vi "Test Clahe Mono Array.vi"(8 "error in (no error)":errorcluster, 11 "Test Case In":refnum<class "01_Image.lvclass">) -> (0 "error out":errorcluster, 3 "Test Case Out":refnum<class "01_Image.lvclass">)   [LabVIEW 2020, in "test.lvlib" / "01_Image.lvclass"]
uses:
  01_Image.lvclass
  4993e8ee-a06a-463a-9684-69129f64d5ce.vi
  image/CLAHE/CLAHE.lvclass
  image/image.lvlib
  image/New Image (Greyscale Preallocated).vi
panel:
  out "data value":u8[][](array[numeric])
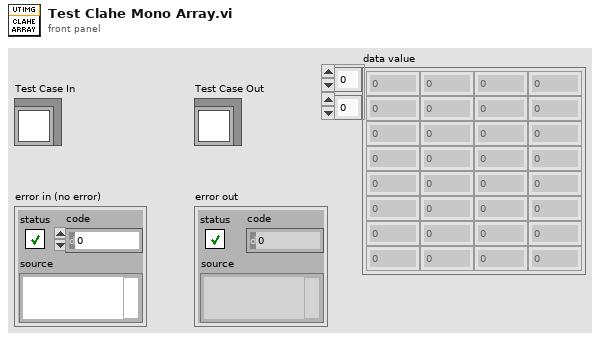
[diagram p1: front panel]
types:
  T1 = typedef "image.lvlib/Greyscale Image.ctl" = refnum<data-value>
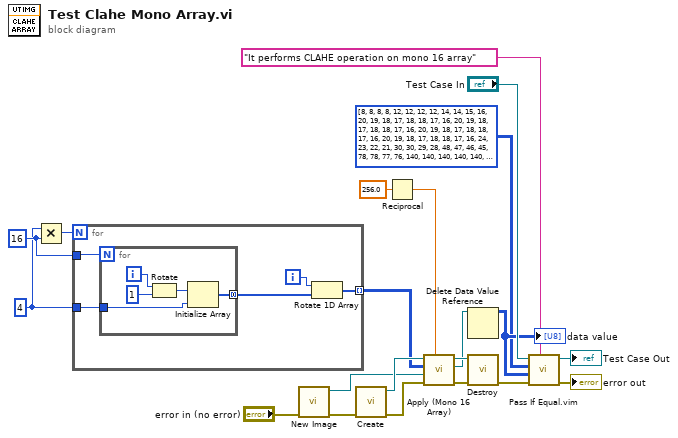
[diagram p0: block diagram]
diagram:
  w8 = 4 ("dimension size")
  w10 = 16
  n1 = Multiply(x=w8, y=w10) -> (x*y=w9:i32)
  n2 = for {
    N: w9 -> [_]
    tunnel: [w24] -> w7 mode=indexing
    tunnel: w10 -> [w23]
    tunnel: w8 -> [w22]
    i -> [w25]
    n3 = for {
      N: w23 -> [_]
      tunnel: [w28] -> w26 mode=concatenating
      tunnel: w22 -> [w27]
      i -> [w31]
      n4 = Rotate(1:u16 1 ("x"), 2:w31) -> (0:w29:u16)
      n5 = Initialize Array(w29, w27) -> (w28:u16[])
    }
    n6 = Rotate 1D Array(1:w26, 2:w25) -> (0:w24:u16[])
  }
  n7 = call-poly "New Image.vi"("error in (no error)"="error in (no error)") -> ("error out"=w15:errorcluster, "Greyscale Image"=w16:T1)  [unwired: 9 in]
  n8 = call "Create.vi"("error in (no error)"=w15) -> ("error out"=w14:errorcluster, "CLAHE"=w18:refnum<class "CLAHE.lvclass">)  [unwired: 9 in]
  n9 = Reciprocal(x=256.0 ("Scaling Factor (Default 1/256)")) -> (1/x=w1:dbl)
  n10 = call "Apply (Mono 16 Array).vi"("Scaling Factor (Default 1/256)"=w1, "error in (no error)"=w14, "Destination Image in"=w16, "Mono 16 Image Data"=w7, "CLAHE in"=w18) -> ("error out"=w13:errorcluster, "Destination Image"=w4:T1, "CLAHE"=w17:refnum<class "CLAHE.lvclass">)  [unwired: 4 in]
  n11 = Delete Data Value Reference(data value reference=w4) -> (data value=w3:u8[][])  [unwired: 1 in, 1 out]
  "data value" <- w3
  n12 = call "Destroy.vi"("error in (no error)"=w13, "CLAHE"=w17) -> ("error out"=w12:errorcluster)  [unwired: 9 in]
  n13 = call "Pass If Equal.vim"("Description"="It performs CLAHE operation on mono 16 array", "error in (no error)"=w12, "Actual"=w3, "Expected"=u8[][] [[8, 8, 8, 8, 12, 12, 12, 12, 14, 14, 15, 16, 20, 19, 18, 17, 18, 18, 17, 16, 20, 19, 18, 17, 18, 18, 17, 16, 20, 19, 18, 17, 18, 18, 17, 16, 20, 19, 18, 17, 18, 18, 17, 16, 24, 23, 22, 21, 30, 30, 29, 28, 48, 47, 46, 45, 78, 78, 77, 76, 140, 140, 140, 140], [140, 8, 8, 8, 8, 12, 12, 12, 12, 14, 15, 16, 16, 19, 18, 17, 16, 18, 17, 16, 16, 19, 18, 17, 16, 18, 17, 16, 16, 19, 18, 17, 16, 18, 17, 16, 16, 19, 18, 17, 16, 18, 17, 16, 16, 23, 22, 21, 20, 30, 29, 28, 28, 47, 46, 45, 44, 78, 77, 76, 76, 140, 140, 140], [140, 140, 8, 8, 8, 8, 12, 12, 12, 12, 15, 16, 16, 15, 18, 17, 16, 15, 17, 16, 16, 15, 18, 17, 16, 15, 17, 16, 16, 15, 18, 17, 16, 15, 17, 16, 16, 15, 18, 17, 16, 15, 17, 16, 16, 15, 22, 21, 20, 19, 29, 28, 28, 27, 46, 45, 44, 43, 77, 76, 76, 76, 140, 140], [140, 140, 140, 8, 8, 8, 8, 12, 12, 12, 12, 16, 16, 15, 14, 17, 16, 15, 14, 16, 16, 15, 14, 17, 16, 15, 14, 16, 16, 15, 14, 17, 16, 15, 14, 16, 16, 15, 14, 17, 16, 15, 14, 16, 16, 15, 14, 21, 20, 19, 18, 28, 28, 27, 26, 45, 44, 43, 42, 76, 76, 76, 76, 140], [140, 140, 140, 140, 8, 8, 8, 8, 12, 12, 12, 12, 16, 15, 14, 13, 16, 15, 14, 13, 16, 15, 14, 13, 16, 15, 14, 13, 16, 15, 14, 13, 16, 15, 14, 13, 16, 15, 14, 13, 16, 15, 14, 13, 16, 15, 14, 13, 20, 19, 18, 17, 28, 27, 26, 25, 44, 43, 42, 41, 76, 76, 76, 76], [76, 140, 140, 140, 140, 8, 8, 8, 8, 12, 12, 12, 12, 15, 14, 13, 12, 15, 14, 14, 13, 16, 15, 14, 13, 16, 15, 14, 13, 16, 15, 14, 13, 16, 15, 14, 13, 16, 15, 14, 13, 16, 15, 14, 13, 16, 15, 14, 13, 20, 19, 18, 17, 28, 27, 26, 25, 44, 43, 42, 41, 76, 76, 76], [76, 76, 140, 140, 140, 140, 7, 7, 8, 8, 12, 12, 12, 11, 14, 13, 12, 12, 15, 14, 14, 13, 15, 14, 14, 13, 16, 15, 14, 13, 15, 14, 14, 13, 16, 15, 14, 13, 15, 14, 14, 13, 16, 15, 14, 13, 15, 14, 14, 13, 20, 19, 18, 17, 27, 26, 26, 25, 44, 43, 42, 42, 77, 77], [76, 76, 76, 140, 140, 140, 140, 7, 7, 7, 8, 12, 12, 11, 11, 13, 13, 12, 12, 15, 15, 14, 13, 15, 14, 13, 13, 16, 15, 14, 13, 15, 14, 13, 13, 16, 15, 14, 13, 15, 14, 13, 13, 16, 15, 14, 13, 15, 14, 13, 13, 20, 19, 18, 17, 27, 26, 25, 25, 44, 43, 43, 43, 78], [76, 76, 76, 76, 140, 140, 140, 140, 7, 7, 8, 8, 12, 12, 11, 10, 13, 13, 12, 12, 16, 15, 14, 13, 15, 14, 14, 13, 16, 15, 14, 13, 15, 14, 14, 13, 16, 15, 14, 13, 15, 14, 14, 13, 16, 15, 14, 13, 15, 14, 14, 13, 20, 19, 18, 17, 27, 26, 26, 25, 44, 44, 44, 44], [40, 76, 76, 76, 76, 140, 140, 140, 140, 7, 7, 8, 8, 12, 11, 11, 10, 13, 13, 13, 13, 16, 15, 14, 13, 15, 14, 14, 13, 16, 15, 14, 13, 15, 14, 14, 13, 16, 15, 14, 13, 15, 14, 14, 13, 16, 15, 14, 13, 15, 14, 14, 13, 20, 19, 18, 17, 27, 26, 26, 25, 45, 45, 45], [40, 40, 76, 76, 76, 76, 140, 140, 140, 140, 7, 8, 8, 8, 12, 11, 11, 11, 14, 14, 14, 13, 16, 15, 14, 13, 15, 15, 14, 13, 16, 15, 14, 13, 15, 15, 14, 13, 16, 15, 14, 13, 15, 15, 14, 13, 16, 15, 14, 13, 15, 15, 14, 13, 20, 19, 18, 17, 27, 27, 26, 26, 46, 46], [40, 40, 40, 76, 76, 76, 76, 140, 140, 140, 140, 8, 8, 8, 8, 12, 12, 11, 11, 15, 15, 14, 13, 16, 15, 14, 13, 16, 15, 14, 13, 16, 15, 14, 13, 16, 15, 14, 13, 16, 15, 14, 13, 16, 15, 14, 13, 16, 15, 14, 13, 16, 15, 14, 13, 20, 19, 18, 17, 28, 27, 27, 27, 47], [40, 40, 40, 40, 76, 76, 76, 76, 140, 140, 140, 140, 8, 8, 8, 8, 12, 12, 12, 12, 16, 15, 14, 13, 16, 15, 14, 13, 16, 15, 14, 13, 16, 15, 14, 13, 16, 15, 14, 13, 16, 15, 14, 13, 16, 15, 14, 13, 16, 15, 14, 13, 16, 15, 14, 13, 20, 19, 18, 17, 28, 28, 28, 28], [21, 41, 41, 41, 41, 76, 76, 76, 76, 140, 140, 140, 140, 8, 8, 8, 8, 12, 12, 12, 12, 15, 14, 13, 12, 15, 14, 14, 13, 16, 15, 14, 13, 16, 15, 14, 13, 16, 15, 14, 13, 16, 15, 14, 13, 16, 15, 14, 13, 16, 15, 14, 13, 16, 15, 14, 13, 20, 19, 18, 17, 28, 28, 28], [22, 22, 42, 42, 42, 42, 77, 77, 76, 76, 140, 140, 140, 140, 7, 7, 8, 8, 12, 12, 12, 11, 14, 13, 12, 12, 15, 14, 14, 13, 15, 14, 14, 13, 16, 15, 14, 13, 15, 14, 14, 13, 16, 15, 14, 13, 15, 14, 14, 13, 16, 15, 14, 13, 15, 14, 14, 13, 20, 19, 18, 18, 29, 29], [23, 23, 23, 43, 43, 43, 42, 77, 77, 77, 76, 140, 140, 140, 140, 7, 7, 7, 8, 12, 12, 11, 11, 13, 13, 12, 12, 15, 15, 14, 13, 15, 14, 13, 13, 16, 15, 14, 13, 15, 14, 13, 13, 16, 15, 14, 13, 15, 14, 13, 13, 16, 15, 14, 13, 15, 14, 13, 13, 20, 19, 19, 19, 30], [24, 24, 24, 24, 44, 44, 43, 42, 77, 77, 76, 76, 140, 140, 140, 140, 7, 7, 8, 8, 12, 12, 11, 10, 13, 13, 12, 12, 16, 15, 14, 13, 15, 14, 14, 13, 16, 15, 14, 13, 15, 14, 14, 13, 16, 15, 14, 13, 15, 14, 14, 13, 16, 15, 14, 13, 15, 14, 14, 13, 20, 20, 20, 20], [13, 25, 25, 25, 25, 44, 44, 43, 42, 77, 77, 76, 76, 140, 140, 140, 140, 7, 7, 8, 8, 12, 11, 11, 10, 13, 13, 13, 13, 16, 15, 14, 13, 15, 14, 14, 13, 16, 15, 14, 13, 15, 14, 14, 13, 16, 15, 14, 13, 15, 14, 14, 13, 16, 15, 14, 13, 15, 14, 14, 13, 21, 21, 21], [14, 14, 26, 26, 26, 25, 44, 44, 43, 42, 77, 76, 76, 76, 140, 140, 140, 140, 7, 8, 8, 8, 12, 11, 11, 11, 14, 14, 14, 13, 16, 15, 14, 13, 15, 15, 14, 13, 16, 15, 14, 13, 15, 15, 14, 13, 16, 15, 14, 13, 15, 15, 14, 13, 16, 15, 14, 13, 15, 15, 14, 14, 22, 22], [15, 15, 15, 27, 27, 26, 25, 44, 44, 43, 42, 76, 76, 76, 76, 140, 140, 140, 140, 8, 8, 8, 8, 12, 12, 11, 11, 15, 15, 14, 13, 16, 15, 14, 13, 16, 15, 14, 13, 16, 15, 14, 13, 16, 15, 14, 13, 16, 15, 14, 13, 16, 15, 14, 13, 16, 15, 14, 13, 16, 15, 15, 15, 23], [16, 16, 16, 16, 28, 27, 26, 25, 44, 43, 42, 41, 76, 76, 76, 76, 140, 140, 140, 140, 8, 8, 8, 8, 12, 12, 12, 12, 16, 15, 14, 13, 16, 15, 14, 13, 16, 15, 14, 13, 16, 15, 14, 13, 16, 15, 14, 13, 16, 15, 14, 13, 16, 15, 14, 13, 16, 15, 14, 13, 16, 16, 16, 16], [9, 17, 17, 17, 17, 28, 27, 26, 25, 44, 43, 42, 41, 76, 76, 76, 76, 140, 140, 140, 140, 8, 8, 8, 8, 12, 12, 12, 12, 15, 14, 13, 12, 15, 14, 14, 13, 16, 15, 14, 13, 16, 15, 14, 13, 16, 15, 14, 13, 16, 15, 14, 13, 16, 15, 14, 13, 16, 15, 14, 13, 16, 16, 16], [10, 10, 18, 18, 18, 17, 27, 26, 26, 25, 44, 43, 42, 42, 77, 77, 76, 76, 140, 140, 140, 140, 7, 7, 8, 8, 12, 12, 12, 11, 14, 13, 12, 12, 15, 14, 14, 13, 15, 14, 14, 13, 16, 15, 14, 13, 15, 14, 14, 13, 16, 15, 14, 13, 15, 14, 14, 13, 16, 15, 14, 14, 17, 17], [11, 11, 11, 19, 19, 18, 17, 27, 26, 25, 25, 44, 43, 43, 42, 77, 77, 77, 76, 140, 140, 140, 140, 7, 7, 7, 8, 12, 12, 11, 11, 13, 13, 12, 12, 15, 15, 14, 13, 15, 14, 13, 13, 16, 15, 14, 13, 15, 14, 13, 13, 16, 15, 14, 13, 15, 14, 13, 13, 16, 15, 15, 15, 18], [12, 12, 12, 12, 20, 19, 18, 17, 27, 26, 26, 25, 44, 44, 43, 42, 77, 77, 76, 76, 140, 140, 140, 140, 7, 7, 8, 8, 12, 12, 11, 10, 13, 13, 12, 12, 16, 15, 14, 13, 15, 14, 14, 13, 16, 15, 14, 13, 15, 14, 14, 13, 16, 15, 14, 13, 15, 14, 14, 13, 16, 16, 16, 16], [9, 13, 13, 13, 13, 20, 19, 18, 17, 27, 26, 26, 25, 44, 44, 43, 42, 77, 77, 76, 76, 140, 140, 140, 140, 7, 7, 8, 8, 12, 11, 11, 10, 13, 13, 13, 13, 16, 15, 14, 13, 15, 14, 14, 13, 16, 15, 14, 13, 15, 14, 14, 13, 16, 15, 14, 13, 15, 14, 14, 13, 17, 17, 17], [10, 10, 14, 14, 14, 13, 20, 19, 18, 17, 27, 27, 26, 25, 44, 44, 43, 42, 77, 76, 76, 76, 140, 140, 140, 140, 7, 8, 8, 8, 12, 11, 11, 11, 14, 14, 14, 13, 16, 15, 14, 13, 15, 15, 14, 13, 16, 15, 14, 13, 15, 15, 14, 13, 16, 15, 14, 13, 15, 15, 14, 14, 18, 18], [11, 11, 11, 15, 15, 14, 13, 20, 19, 18, 17, 28, 27, 26, 25, 44, 44, 43, 42, 76, 76, 76, 76, 140, 140, 140, 140, 8, 8, 8, 8, 12, 12, 11, 11, 15, 15, 14, 13, 16, 15, 14, 13, 16, 15, 14, 13, 16, 15, 14, 13, 16, 15, 14, 13, 16, 15, 14, 13, 16, 15, 15, 15, 19], [12, 12, 12, 12, 16, 15, 14, 13, 20, 19, 18, 17, 28, 27, 26, 25, 44, 43, 42, 41, 76, 76, 76, 76, 140, 140, 140, 140, 8, 8, 8, 8, 12, 12, 12, 12, 16, 15, 14, 13, 16, 15, 14, 13, 16, 15, 14, 13, 16, 15, 14, 13, 16, 15, 14, 13, 16, 15, 14, 13, 16, 16, 16, 16], [9, 13, 13, 13, 13, 16, 15, 14, 13, 20, 19, 18, 17, 28, 27, 26, 25, 44, 43, 42, 41, 76, 76, 76, 76, 140, 140, 140, 140, 8, 8, 8, 8, 12, 12, 12, 12, 15, 14, 13, 12, 15, 14, 14, 13, 16, 15, 14, 13, 16, 15, 14, 13, 16, 15, 14, 13, 16, 15, 14, 13, 16, 16, 16], [10, 10, 14, 14, 14, 13, 15, 14, 14, 13, 20, 19, 18, 17, 27, 26, 26, 25, 44, 43, 42, 42, 77, 77, 76, 76, 140, 140, 140, 140, 7, 7, 8, 8, 12, 12, 12, 11, 14, 13, 12, 12, 15, 14, 14, 13, 15, 14, 14, 13, 16, 15, 14, 13, 15, 14, 14, 13, 16, 15, 14, 14, 17, 17], [11, 11, 11, 15, 15, 14, 13, 15, 14, 13, 13, 20, 19, 18, 17, 27, 26, 25, 25, 44, 43, 43, 42, 77, 77, 77, 76, 140, 140, 140, 140, 7, 7, 7, 8, 12, 12, 11, 11, 13, 13, 12, 12, 15, 15, 14, 13, 15, 14, 13, 13, 16, 15, 14, 13, 15, 14, 13, 13, 16, 15, 15, 15, 18], [12, 12, 12, 12, 16, 15, 14, 13, 15, 14, 14, 13, 20, 19, 18, 17, 27, 26, 26, 25, 44, 44, 43, 42, 77, 77, 76, 76, 140, 140, 140, 140, 7, 7, 8, 8, 12, 12, 11, 10, 13, 13, 12, 12, 16, 15, 14, 13, 15, 14, 14, 13, 16, 15, 14, 13, 15, 14, 14, 13, 16, 16, 16, 16], [9, 13, 13, 13, 13, 16, 15, 14, 13, 15, 14, 14, 13, 20, 19, 18, 17, 27, 26, 26, 25, 44, 44, 43, 42, 77, 77, 76, 76, 140, 140, 140, 140, 7, 7, 8, 8, 12, 11, 11, 10, 13, 13, 13, 13, 16, 15, 14, 13, 15, 14, 14, 13, 16, 15, 14, 13, 15, 14, 14, 13, 17, 17, 17], [10, 10, 14, 14, 14, 13, 16, 15, 14, 13, 15, 15, 14, 13, 20, 19, 18, 17, 27, 27, 26, 25, 44, 44, 43, 42, 77, 76, 76, 76, 140, 140, 140, 140, 7, 8, 8, 8, 12, 11, 11, 11, 14, 14, 14, 13, 16, 15, 14, 13, 15, 15, 14, 13, 16, 15, 14, 13, 15, 15, 14, 14, 18, 18], [11, 11, 11, 15, 15, 14, 13, 16, 15, 14, 13, 16, 15, 14, 13, 20, 19, 18, 17, 28, 27, 26, 25, 44, 44, 43, 42, 76, 76, 76, 76, 140, 140, 140, 140, 8, 8, 8, 8, 12, 12, 11, 11, 15, 15, 14, 13, 16, 15, 14, 13, 16, 15, 14, 13, 16, 15, 14, 13, 16, 15, 15, 15, 19], [12, 12, 12, 12, 16, 15, 14, 13, 16, 15, 14, 13, 16, 15, 14, 13, 20, 19, 18, 17, 28, 27, 26, 25, 44, 43, 42, 41, 76, 76, 76, 76, 140, 140, 140, 140, 8, 8, 8, 8, 12, 12, 12, 12, 16, 15, 14, 13, 16, 15, 14, 13, 16, 15, 14, 13, 16, 15, 14, 13, 16, 16, 16, 16], [9, 13, 13, 13, 13, 16, 15, 14, 13, 16, 15, 14, 13, 16, 15, 14, 13, 20, 19, 18, 17, 28, 27, 26, 25, 44, 43, 42, 41, 76, 76, 76, 76, 140, 140, 140, 140, 8, 8, 8, 8, 12, 12, 12, 12, 15, 14, 13, 12, 15, 14, 14, 13, 16, 15, 14, 13, 16, 15, 14, 13, 16, 16, 16], [10, 10, 14, 14, 14, 13, 15, 14, 14, 13, 16, 15, 14, 13, 15, 14, 14, 13, 20, 19, 18, 17, 27, 26, 26, 25, 44, 43, 42, 42, 77, 77, 76, 76, 140, 140, 140, 140, 7, 7, 8, 8, 12, 12, 12, 11, 14, 13, 12, 12, 15, 14, 14, 13, 15, 14, 14, 13, 16, 15, 14, 14, 17, 17], [11, 11, 11, 15, 15, 14, 13, 15, 14, 13, 13, 16, 15, 14, 13, 15, 14, 13, 13, 20, 19, 18, 17, 27, 26, 25, 25, 44, 43, 43, 42, 77, 77, 77, 76, 140, 140, 140, 140, 7, 7, 7, 8, 12, 12, 11, 11, 13, 13, 12, 12, 15, 15, 14, 13, 15, 14, 13, 13, 16, 15, 15, 15, 18], [12, 12, 12, 12, 16, 15, 14, 13, 15, 14, 14, 13, 16, 15, 14, 13, 15, 14, 14, 13, 20, 19, 18, 17, 27, 26, 26, 25, 44, 44, 43, 42, 77, 77, 76, 76, 140, 140, 140, 140, 7, 7, 8, 8, 12, 12, 11, 10, 13, 13, 12, 12, 16, 15, 14, 13, 15, 14, 14, 13, 16, 16, 16, 16], [9, 13, 13, 13, 13, 16, 15, 14, 13, 15, 14, 14, 13, 16, 15, 14, 13, 15, 14, 14, 13, 20, 19, 18, 17, 27, 26, 26, 25, 44, 44, 43, 42, 77, 77, 76, 76, 140, 140, 140, 140, 7, 7, 8, 8, 12, 11, 11, 10, 13, 13, 13, 13, 16, 15, 14, 13, 15, 14, 14, 13, 17, 17, 17], [10, 10, 14, 14, 14, 13, 16, 15, 14, 13, 15, 15, 14, 13, 16, 15, 14, 13, 15, 15, 14, 13, 20, 19, 18, 17, 27, 27, 26, 25, 44, 44, 43, 42, 77, 76, 76, 76, 140, 140, 140, 140, 7, 8, 8, 8, 12, 11, 11, 11, 14, 14, 14, 13, 16, 15, 14, 13, 15, 15, 14, 14, 18, 18], [11, 11, 11, 15, 15, 14, 13, 16, 15, 14, 13, 16, 15, 14, 13, 16, 15, 14, 13, 16, 15, 14, 13, 20, 19, 18, 17, 28, 27, 26, 25, 44, 44, 43, 42, 76, 76, 76, 76, 140, 140, 140, 140, 8, 8, 8, 8, 12, 12, 11, 11, 15, 15, 14, 13, 16, 15, 14, 13, 16, 15, 15, 15, 19], [12, 12, 12, 12, 16, 15, 14, 13, 16, 15, 14, 13, 16, 15, 14, 13, 16, 15, 14, 13, 16, 15, 14, 13, 20, 19, 18, 17, 28, 27, 26, 25, 44, 43, 42, 41, 76, 76, 76, 76, 140, 140, 140, 140, 8, 8, 8, 8, 12, 12, 12, 12, 16, 15, 14, 13, 16, 15, 14, 13, 16, 16, 16, 16], [9, 13, 13, 13, 13, 16, 15, 14, 13, 16, 15, 14, 13, 16, 15, 14, 13, 16, 15, 14, 13, 16, 15, 14, 13, 20, 19, 18, 17, 28, 27, 26, 25, 44, 43, 42, 41, 76, 76, 76, 76, 140, 140, 140, 140, 8, 8, 8, 8, 12, 12, 12, 12, 15, 14, 13, 12, 15, 14, 14, 13, 16, 16, 16], [10, 10, 14, 14, 14, 13, 15, 14, 14, 13, 16, 15, 14, 13, 15, 14, 14, 13, 16, 15, 14, 13, 15, 14, 14, 13, 20, 19, 18, 17, 27, 26, 26, 25, 44, 43, 42, 42, 77, 77, 76, 76, 140, 140, 140, 140, 7, 7, 8, 8, 12, 12, 12, 11, 14, 13, 12, 12, 15, 14, 14, 14, 17, 17], [11, 11, 11, 15, 15, 14, 13, 15, 14, 13, 13, 16, 15, 14, 13, 15, 14, 13, 13, 16, 15, 14, 13, 15, 14, 13, 13, 20, 19, 18, 17, 27, 26, 25, 25, 44, 43, 43, 42, 77, 77, 77, 76, 140, 140, 140, 140, 7, 7, 7, 8, 12, 12, 11, 11, 13, 13, 12, 12, 15, 15, 15, 15, 18], [12, 12, 12, 12, 16, 15, 14, 13, 15, 14, 14, 13, 16, 15, 14, 13, 15, 14, 14, 13, 16, 15, 14, 13, 15, 14, 14, 13, 20, 19, 18, 17, 27, 26, 26, 25, 44, 44, 43, 42, 77, 77, 76, 76, 140, 140, 140, 140, 7, 7, 8, 8, 12, 12, 11, 10, 13, 13, 12, 12, 16, 16, 16, 16], [9, 13, 13, 13, 13, 16, 15, 14, 13, 15, 14, 14, 13, 16, 15, 14, 13, 15, 14, 14, 13, 16, 15, 14, 13, 15, 14, 14, 13, 20, 19, 18, 17, 27, 26, 26, 25, 44, 44, 43, 42, 77, 77, 76, 76, 140, 140, 140, 140, 7, 7, 8, 8, 12, 11, 11, 10, 13, 13, 13, 13, 17, 17, 17], [10, 10, 14, 14, 14, 13, 16, 15, 14, 13, 15, 15, 14, 13, 16, 15, 14, 13, 15, 15, 14, 13, 16, 15, 14, 13, 15, 15, 14, 13, 20, 19, 18, 17, 27, 27, 26, 25, 44, 44, 43, 42, 77, 76, 76, 76, 140, 140, 140, 140, 7, 8, 8, 8, 12, 11, 11, 11, 14, 14, 14, 14, 18, 18], [11, 11, 11, 15, 15, 14, 13, 16, 15, 14, 13, 16, 15, 14, 13, 16, 15, 14, 13, 16, 15, 14, 13, 16, 15, 14, 13, 16, 15, 14, 13, 20, 19, 18, 17, 28, 27, 26, 25, 44, 44, 43, 42, 76, 76, 76, 76, 140, 140, 140, 140, 8, 8, 8, 8, 12, 12, 11, 11, 15, 15, 15, 15, 19], [12, 12, 12, 12, 16, 15, 14, 13, 16, 15, 14, 13, 16, 15, 14, 13, 16, 15, 14, 13, 16, 15, 14, 13, 16, 15, 14, 13, 16, 15, 14, 13, 20, 19, 18, 17, 28, 27, 26, 25, 44, 43, 42, 41, 76, 76, 76, 76, 140, 140, 140, 140, 8, 8, 8, 8, 12, 12, 12, 12, 16, 16, 16, 16], [9, 13, 13, 13, 13, 16, 15, 14, 13, 16, 15, 14, 13, 16, 15, 14, 13, 16, 15, 14, 13, 16, 15, 14, 13, 16, 15, 14, 13, 16, 15, 14, 13, 20, 19, 18, 17, 28, 27, 26, 25, 44, 43, 42, 41, 76, 76, 76, 76, 140, 140, 140, 140, 8, 8, 8, 8, 12, 12, 12, 12, 16, 16, 16], [10, 10, 14, 14, 14, 13, 15, 14, 14, 13, 16, 15, 14, 13, 15, 14, 14, 13, 16, 15, 14, 13, 15, 14, 14, 13, 16, 15, 14, 13, 15, 14, 14, 13, 20, 19, 18, 17, 27, 26, 26, 25, 44, 43, 42, 42, 77, 77, 76, 76, 140, 140, 140, 140, 7, 7, 8, 8, 12, 12, 12, 12, 15, 15], [11, 11, 11, 15, 15, 14, 13, 15, 14, 13, 13, 16, 15, 14, 13, 15, 14, 13, 13, 16, 15, 14, 13, 15, 14, 13, 13, 16, 15, 14, 13, 15, 14, 13, 13, 20, 19, 18, 17, 27, 26, 25, 25, 44, 43, 43, 42, 77, 77, 77, 76, 140, 140, 140, 140, 7, 7, 7, 8, 12, 12, 12, 12, 14], [12, 12, 12, 12, 16, 15, 14, 13, 15, 14, 14, 13, 16, 15, 14, 13, 15, 14, 14, 13, 16, 15, 14, 13, 15, 14, 14, 13, 16, 15, 14, 13, 15, 14, 14, 13, 20, 19, 18, 17, 27, 26, 26, 25, 44, 44, 43, 42, 77, 77, 76, 76, 140, 140, 140, 140, 7, 7, 8, 8, 12, 12, 12, 12], [9, 13, 13, 13, 13, 16, 15, 14, 13, 15, 14, 14, 13, 16, 15, 14, 13, 15, 14, 14, 13, 16, 15, 14, 13, 15, 14, 14, 13, 16, 15, 14, 13, 15, 14, 14, 13, 20, 19, 18, 17, 27, 26, 26, 25, 44, 44, 43, 42, 77, 77, 76, 76, 140, 140, 140, 140, 7, 7, 8, 8, 12, 12, 12], [10, 10, 14, 14, 14, 13, 16, 15, 14, 13, 15, 15, 14, 13, 16, 15, 14, 13, 15, 15, 14, 13, 16, 15, 14, 13, 15, 15, 14, 13, 16, 15, 14, 13, 15, 15, 14, 13, 20, 19, 18, 17, 27, 27, 26, 25, 44, 44, 43, 42, 77, 76, 76, 76, 140, 140, 140, 140, 7, 8, 8, 8, 12, 12], [11, 11, 11, 15, 15, 14, 13, 16, 15, 14, 13, 16, 15, 14, 13, 16, 15, 14, 13, 16, 15, 14, 13, 16, 15, 14, 13, 16, 15, 14, 13, 16, 15, 14, 13, 16, 15, 14, 13, 20, 19, 18, 17, 28, 27, 26, 25, 44, 44, 43, 42, 76, 76, 76, 76, 140, 140, 140, 140, 8, 8, 8, 8, 12], [12, 12, 12, 12, 16, 15, 14, 13, 16, 15, 14, 13, 16, 15, 14, 13, 16, 15, 14, 13, 16, 15, 14, 13, 16, 15, 14, 13, 16, 15, 14, 13, 16, 15, 14, 13, 16, 15, 14, 13, 20, 19, 18, 17, 28, 27, 26, 25, 44, 43, 42, 41, 76, 76, 76, 76, 140, 140, 140, 140, 8, 8, 8, 8], [8, 12, 12, 12, 12, 15, 14, 13, 12, 15, 14, 13, 12, 15, 14, 13, 12, 15, 14, 13, 12, 15, 14, 13, 12, 15, 14, 13, 12, 15, 14, 13, 12, 15, 14, 13, 12, 15, 14, 13, 12, 19, 18, 17, 16, 27, 26, 25, 24, 43, 42, 41, 40, 76, 76, 76, 76, 140, 140, 140, 140, 8, 8, 8], [8, 8, 12, 12, 12, 11, 14, 13, 12, 11, 14, 13, 12, 11, 14, 13, 12, 11, 14, 13, 12, 11, 14, 13, 12, 11, 14, 13, 12, 11, 14, 13, 12, 11, 14, 13, 12, 11, 14, 13, 12, 11, 18, 17, 16, 15, 26, 25, 24, 23, 42, 41, 40, 40, 76, 76, 76, 76, 140, 140, 140, 140, 8, 8], [8, 8, 8, 12, 12, 11, 10, 13, 12, 11, 10, 13, 12, 11, 10, 13, 12, 11, 10, 13, 12, 11, 10, 13, 12, 11, 10, 13, 12, 11, 10, 13, 12, 11, 10, 13, 12, 11, 10, 13, 12, 11, 10, 17, 16, 15, 14, 25, 24, 23, 22, 41, 40, 40, 40, 76, 76, 76, 76, 140, 140, 140, 140, 8]] ("data value"), "LUnit Test Case In"="Test Case In") -> ("error out"=→"error out":errorcluster, "LUnit Test Case Out"=→"Test Case Out":refnum<class "01_Image.lvclass">)  [unwired: 5 in]
